vi "GetStandardEventStatusRegister.vi"(8 "Error In":errorcluster, 11 "Keithley 7001 In":refnum<visa-resource-name>) -> (0 "Error Out":errorcluster, 2 "Status Event Register":bool[](array[boolean]), 3 "Keithley 7001 Out":refnum<visa-resource-name>)   [LabVIEW 2012, in "Keithley-7001.lvlib"]
uses:
  Keithley-7001.lvlib
panel:
  # "OPC"
  # "EXE"
  # "URQ"
  # "QYE"
  # "PON"
  # "DDE"
  # "CME"
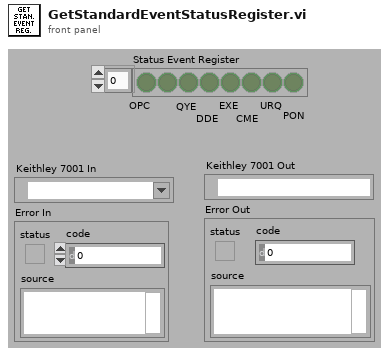
[diagram p1: front panel]
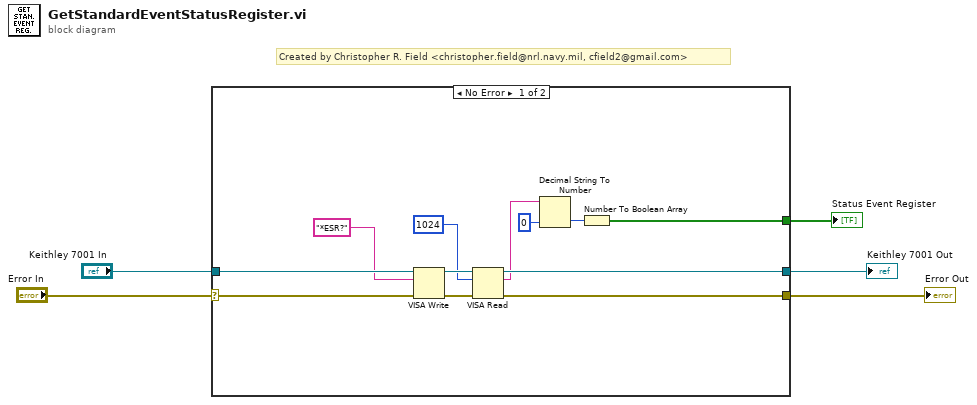
[diagram p0: block diagram]
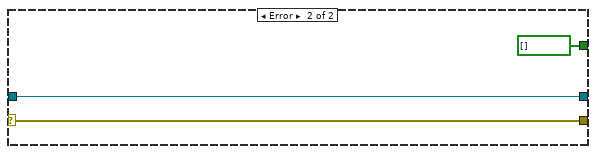
[diagram p2: hidden frame]
diagram:
  # "Created by Christopher R. Field <christopher.field@nrl.navy.mil, cfield2@gmail.com>"
  n1 = case shown="No Error" "Error In" {
    selector: "Error In" -> [w6 w20]
    tunnel: "Keithley 7001 In" -> [w15 w19]
    tunnel: [w14 w19] -> w4
    tunnel: [w13 w20] -> w3
    tunnel: [w8 bool[] [] ("Boolean array")] -> w2
    frame No Error {
      n2 = VISA Write(VISA resource name=w15, write buffer="*ESR?", error in (no error)=w6) -> (VISA resource name out=w17:refnum<visa-resource-name>, error out=w16:errorcluster)  [unwired: 1 out]
      n3 = VISA Read(VISA resource name=w17, byte count=u32 1024, error in (no error)=w16) -> (VISA resource name out=w14:refnum<visa-resource-name>, read buffer=w11:string, error out=w13:errorcluster)  [unwired: 1 out]
      n4 = Decimal String To Number(string=w11, default (0L)=u16 0 ("default (0 I32)")) -> (number=w9:u16)  [unwired: 1 in, 1 out]
      n5 = Number To Boolean Array(number=w9) -> (Boolean array=w8:bool[])
    }
    frame Error {
    }
  }
  "Keithley 7001 Out" <- w4
  "Error Out" <- w3
  "Status Event Register" <- w2
